vi "ConvertVIRPFunctionToString.vi"(11 "Function":T1(ring)) -> (3 "Function":string)   [LabVIEW 2012, in "Keithley-2602.lvlib"]
uses:
  Keithley-2602.lvlib
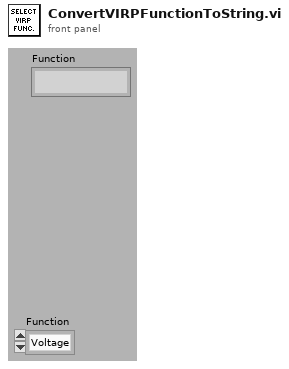
[diagram p1: front panel]
types:
  T1 = enum16{"Voltage", "Current", "Resistance", "Power"}
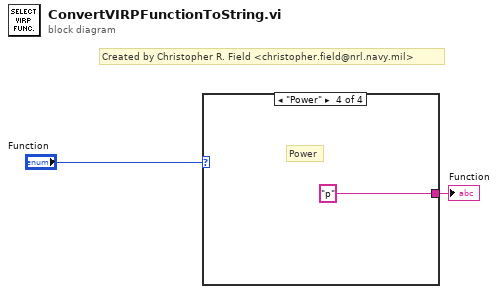
[diagram p0: block diagram]
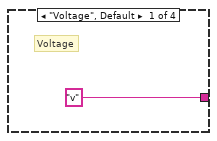
[diagram p2: hidden frame]
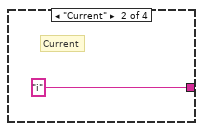
[diagram p3: hidden frame]
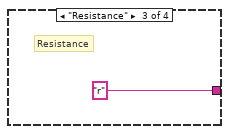
[diagram p4: hidden frame]
diagram:
  # "Created by Christopher R. Field <christopher.field@nrl.navy.mil>"
  n1 = case shown="\"Power\"" "Function" {
    tunnel: ["v" "i" "r" "p"] -> w2
    frame "Voltage", Default {
      # "Voltage"
    }
    frame "Current" {
      # "Current"
    }
    frame "Resistance" {
      # "Resistance"
    }
    frame "Power" {
      # "Power"
    }
  }
  "Function" <- w2
